vi "AudioOut Block Config Pane.vi"(6 "_SubPanelMessages":refnum<notifier>, 9 "_myEmbeddedToFrameEvent":T7, 10 "_myEmbedded.Exit":refnum<user-event>, 11 "-Property Bundle":cluster{"Name":string, "Value":variant}[](array[cluster])) -> (1 "_Connection Informations":T3, 2 "_Scripter Input":T9)   [LabVIEW 2021]
doc: "Writes values to one or more audio output channels on the NI myRIO. Use this Express VI to write multiple samples for each channel at one time."
uses:
  <vilib>/myRIO/Common/Express VI Framework/xctls/myRIO Channel List/myRIO Channel List.xctl
  <vilib>/myRIO/Common/Express VI Framework/typedefs/Config Pane to Framework Ref.ctl
  <vilib>/myRIO/Common/Express VI Framework/typedefs/Data Validate Ref.ctl
  <vilib>/myRIO/Common/Express VI Framework/typedefs/Scripter Input.ctl
  <vilib>/myRIO/Common/Express VI Framework/typedefs/WireThrough Terminal Names.ctl
  <vilib>/myRIO/Common/Express VI Framework/typedefs/Instrument Driver Method Descriptor Array.ctl
  <vilib>/myRIO/Common/Express VI Framework/typedefs/Instrument Driver Method Descriptor.ctl
  <vilib>/myRIO/Common/Express VI Framework/typedefs/Sub Panel Messages.ctl
  <vilib>/myRIO/Common/Express VI Framework/typedefs/Connection Informations.ctl
  <vilib>/myRIO/Common/Instrument Driver Framework/Utilities/typedefs/Channel Types.ctl
  <vilib>/myRIO/Common/Express VI Framework/vis/Express VI Framework Strings Global.vi
panel:
  in  "Sample Rate Unit":string="kHz"
  out "_learnMoreLatency":string="Gaps exist between sequential n samples generations. Learn more"
  out "_learnMoreFrequency":string="Detailed information about valid sample rates for this Express VI. Learn more"
  in  "Wait Until Done?":bool caption="Wait until done?"
  in  "_Validate":bool
  in  "Sample Rate:":dbl=1.0 caption="Sample rate:"
  in  "Name:":string="Audio output (n samples)" caption="Node name:"
  in  "Selected Channel List":T1[](xcontrol)=[{"Channel Name"=0, "Channel Alias"="", "Remove Channel"=FALSE, "Index"=0}, {"Channel Name"=1, "Channel Alias"="", "Remove Channel"=FALSE, "Index"=1}]
  in  "_Default Alias String":string
  in  "_VI Default Name (Edit and make value default)":string="Audio output (n samples)"
  in  "_WireThrough Info (Edit and make value default)":T4={"WireThrough Top In"="AudioOut (N Samples) Ref In", "WireThrough Bottom In"="error in (no error)", "WireThrough Top Out"="AudioOut (N Samples) Ref Out", "WireThrough Bottom Out"="error out"}
  in  "_Template Array (Edit and make value default)":T5=[{"Function Name"="Smart Open", "VI Path"=path "<vilib>/myRIO/Instrument Drivers/Onboard IO/AudioOut Block/vis", "Script"=TRUE, "Inputs"=[{"name"="Channel Names", "value"=variant, "Config Pane Only"=TRUE, "Build Array"=FALSE, "Bundle Cluster"=FALSE, "Show Term"=FALSE, "alias"=[], "Required Input"=FALSE}], "Outputs"=[], "VI Class"=enum."Open", "Controls Refs[]"=[], "Inline"=FALSE}, {"Function Name"="Open", "VI Path"=path "<vilib>/myRIO/Instrument Drivers/Onboard IO/AudioOut Block/vis", "Script"=FALSE, "Inputs"=[{"name"="Channel Names", "value"=variant, "Config Pane Only"=TRUE, "Build Array"=FALSE, "Bundle Cluster"=FALSE, "Show Term"=FALSE, "alias"=[], "Required Input"=FALSE}], "Outputs"=[], "VI Class"=enum."Open", "Controls Refs[]"=[], "Inline"=FALSE}, {"Function Name"="Write", "VI Path"=path "<vilib>/myRIO/Instrument Drivers/Onboard IO/AudioOut Block/vis", "Script"=TRUE, "Inputs"=[{"name"="Values", "value"=variant, "Config Pane Only"=FALSE, "Build Array"=TRUE, "Bundle Cluster"=FALSE, "Show Term"=TRUE, "alias"=[], "Required Input"=TRUE}, {"name"="Sample Rate [Hz]", "value"=variant, "Config Pane Only"=TRUE, "Build Array"=FALSE, "Bundle Cluster"=FALSE, "Show Term"=FALSE, "alias"=[], "Required Input"=FALSE}, {"name"="Wait Until Done?", "value"=variant, "Config Pane Only"=TRUE, "Build Array"=FALSE, "Bundle Cluster"=FALSE, "Show Term"=FALSE, "alias"=[], "Required Input"=FALSE}], "Outputs"=[], "VI Class"=enum."Data", "Controls Refs[]"=[], "Inline"=FALSE}, {"Function Name"="Close", "VI Path"=path "<vilib>/myRIO/Instrument Drivers/Onboard IO/AudioOut Block/vis", "Script"=FALSE, "Inputs"=[], "Outputs"=[], "VI Class"=enum."Close", "Controls Refs[]"=[], "Inline"=FALSE}]
  in  "_Test Close":bool
  # "User Visible Area"
  # "NOTE: Tab Order has been set\nfor this Front Panel.\n1. Name: (string control)\n2. Add Channel (button)\n3. Selected Channel List (array)\n\nAll other controls are excluded \nfrom Tabbing order\n\nTo exlude a control from context\nhelp prefix its label text with a '-'"
  # "kHz"
  # "This Express VI waits until the write operation completes."
  # "Gap:"
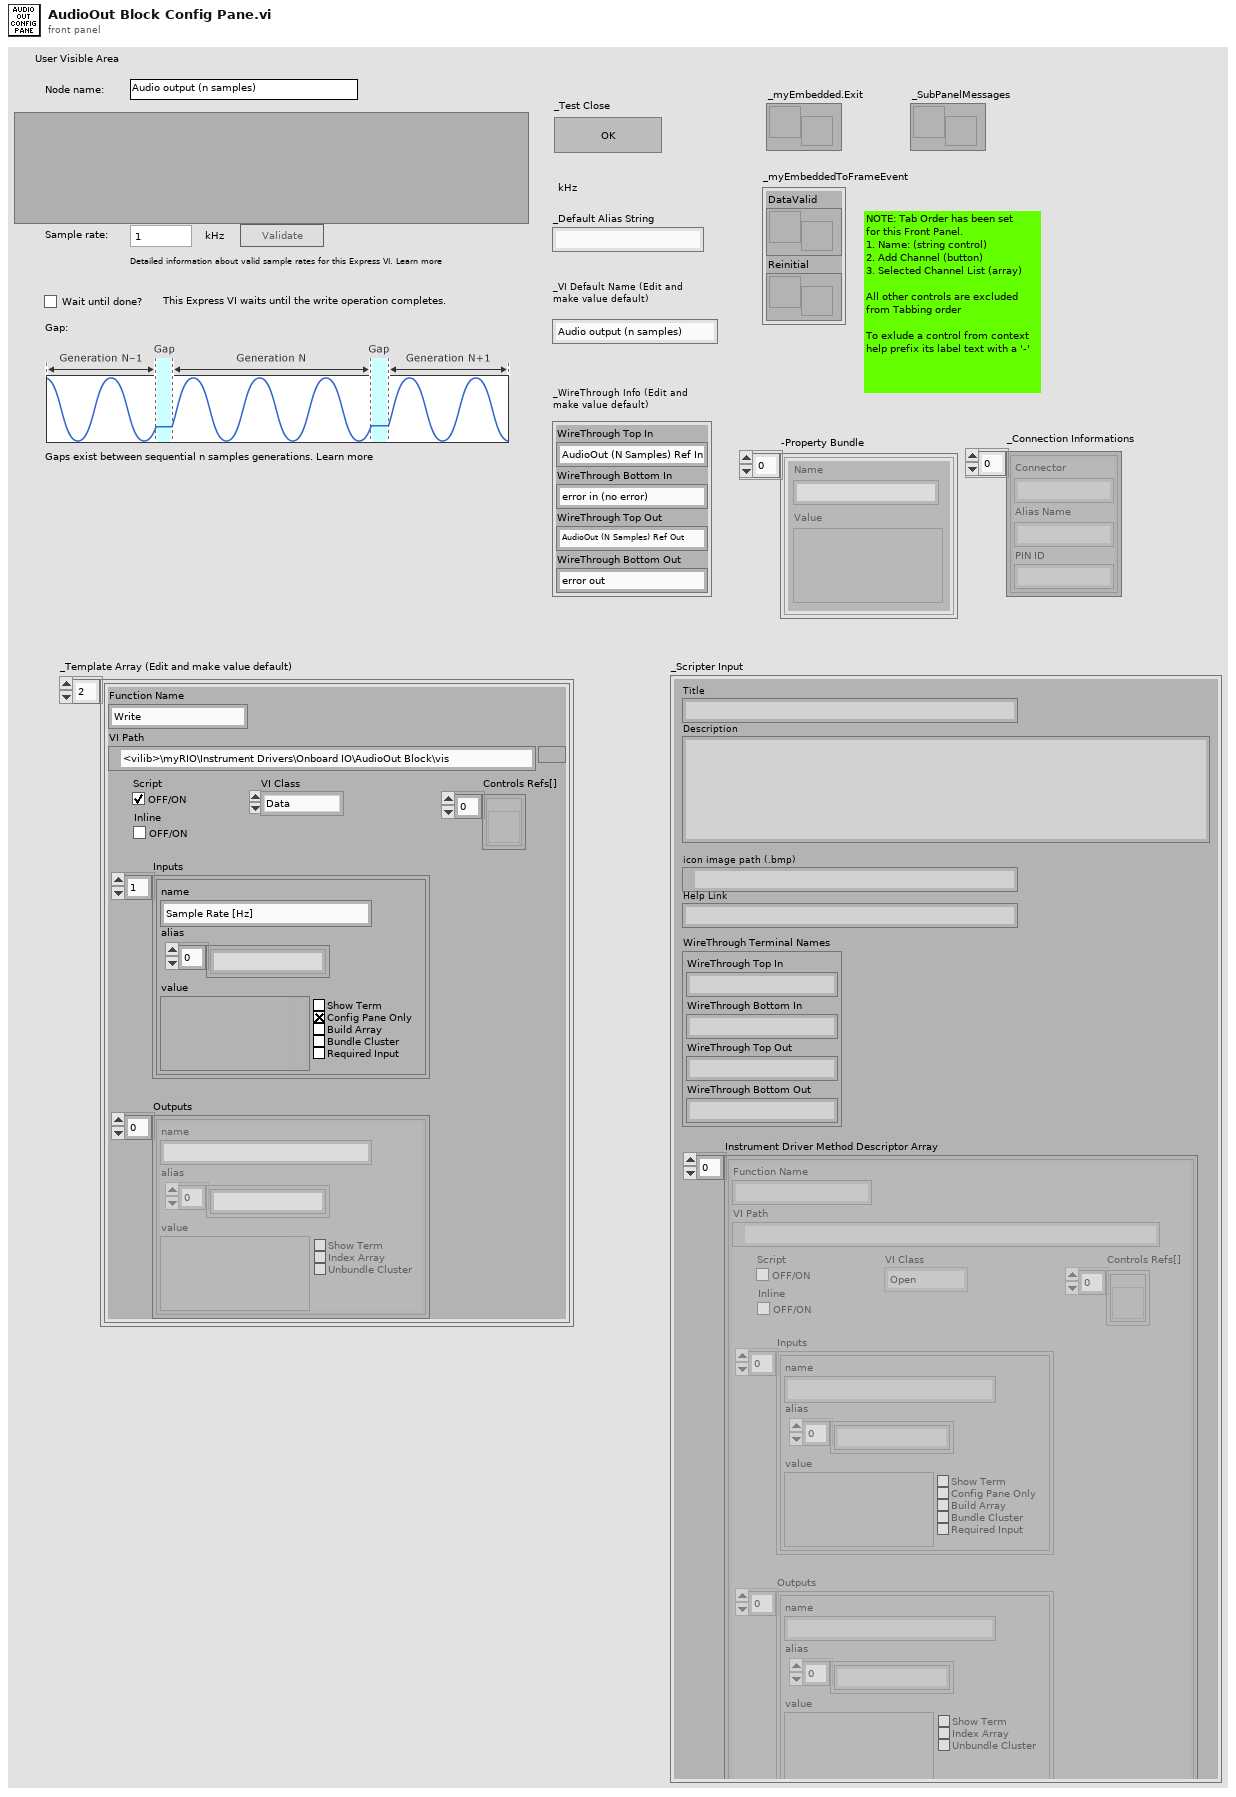
[diagram p1: front panel]
types:
  T1 = typedef "myRIO Channel List.xctl/Channel Data.ctl" = cluster{"Channel Name":u16, "Channel Alias":string, "Remove Channel":T2, "Index":i32}
  T2 = typedef "myRIO Channel List.xctl/Remove Channel.ctl" = bool
  T3 = typedef "Connection Informations.ctl" = cluster{"Connector":string, "Alias Name":string, "PIN ID":string}[]
  T4 = typedef "WireThrough Terminal Names.ctl" = cluster{"WireThrough Top In":string, "WireThrough Bottom In":string, "WireThrough Top Out":string, "WireThrough Bottom Out":string}
  T5 = typedef "Instrument Driver Method Descriptor Array.ctl" = T6[]
  T6 = typedef "Instrument Driver Method Descriptor.ctl" = cluster{"Function Name":string, "VI Path":path, "Script":bool, "Inputs":cluster{"name":string, "value":variant, "Config Pane Only":bool, "Build Array":bool, "Bundle Cluster":bool, "Show Term":bool, "alias":string[], "Required Input":bool}[], "Outputs":cluster{"name":string, "value":variant, "Show Term":bool, "Index Array":bool, "Unbundle Cluster":bool, "alias":string[]}[], "VI Class":enum16{"Open", "Configure", "Data", "Manage", "Close"}, "Controls Refs[]":refnum<vi>[], "Inline":bool}
  T7 = typedef "Config Pane to Framework Ref.ctl" = cluster{"DataValid":T8, "Reinitial":refnum<user-event>}
  T8 = typedef "Data Validate Ref.ctl" = refnum<user-event>
  T9 = typedef "Scripter Input.ctl" = cluster{"Title":string, "Description":string, "icon image path (.bmp)":path, "Help Link":string, "WireThrough Terminal Names":T4, "Instrument Driver Method Descriptor Array":T5}
  T10 = typedef "Channel Types.ctl" = enum32{"Unknown", "AI", "AO", "DIO - DI", "DIO", "DIO - DO", "I2C", "PWM", "Encoder", "SPI", "UART", "Accelerometer", "DIO - LED", "DIO - Button", "AI (N Samples)", "AudioIn (N Samples)", "AO (N Samples)", "AudioOut (N Samples)", "DI (N Samples)", "DO (N Samples)", "AI IRQ", "DI IRQ", "Timer IRQ", "RSL", "Relay", "CAN", "AI (Continuous)", "AO (Continuous)"}
  T11 = typedef "Channel Info.ctl" = cluster{"Channel Name":string, "Alias":string, "Used?":bool, "Not Support?":bool, "Property Bundle":cluster{"Name":string, "Value":variant}[]}
  T12 = typedef "Sub Panel Messages.ctl" = enum16{"Initialized"}
  T13 = enum8{"Enabled", "Disabled", "Disabled and Grayed Out"}
  T14 = cluster{"Connector":string, "Alias Name":string, "PIN ID":string}[]
  T15 = cluster{"name":string, "value":variant, "Config Pane Only":bool, "Build Array":bool, "Bundle Cluster":bool, "Show Term":bool, "alias":string[], "Required Input":bool}[]
  T16 = cluster{"name":string, "value":variant, "Config Pane Only":bool, "Build Array":bool, "Bundle Cluster":bool, "Show Term":bool, "alias":string[], "Required Input":bool}
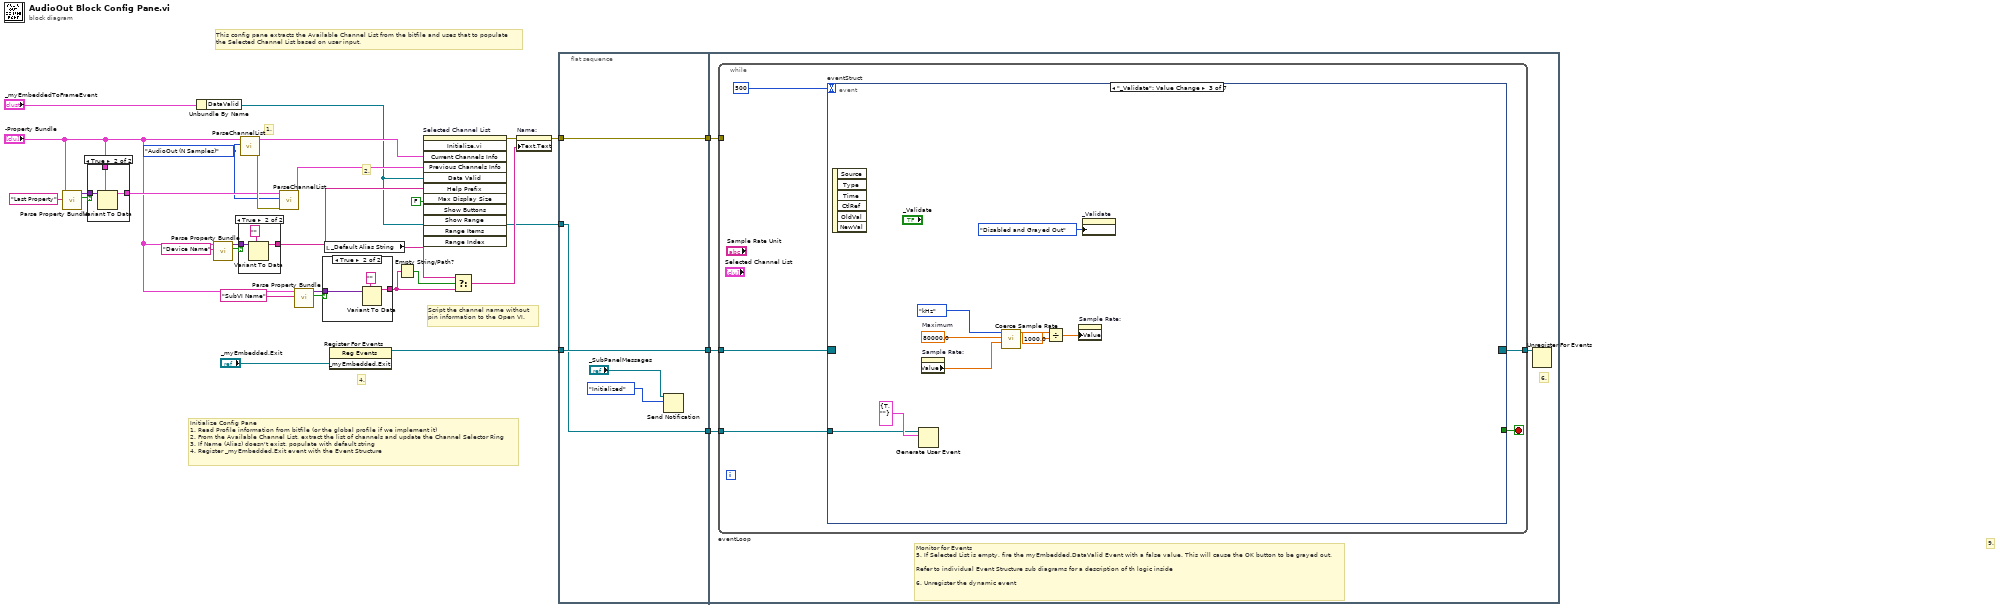
[diagram p0: block diagram]
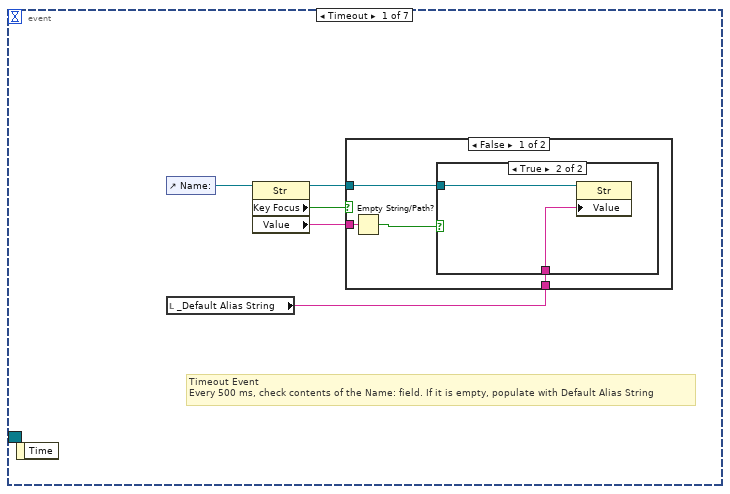
[diagram p2: hidden frame]
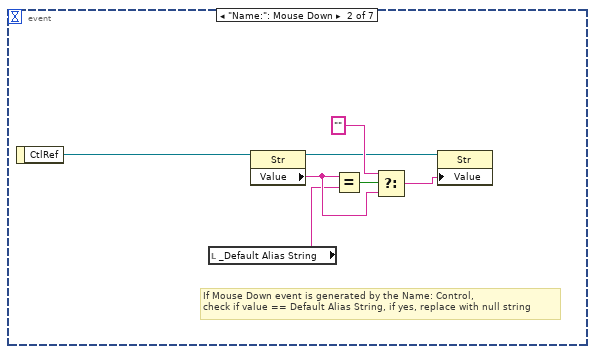
[diagram p5: hidden frame]
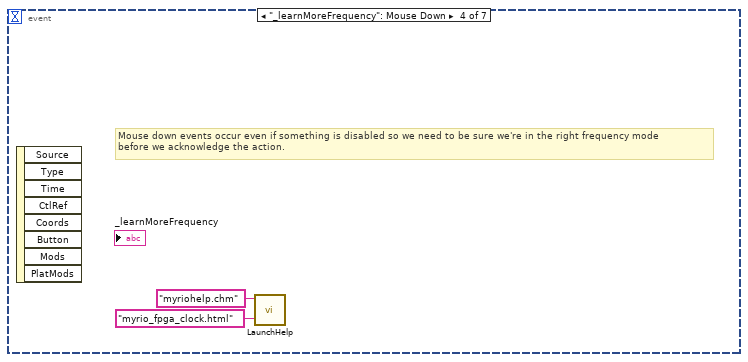
[diagram p6: hidden frame]
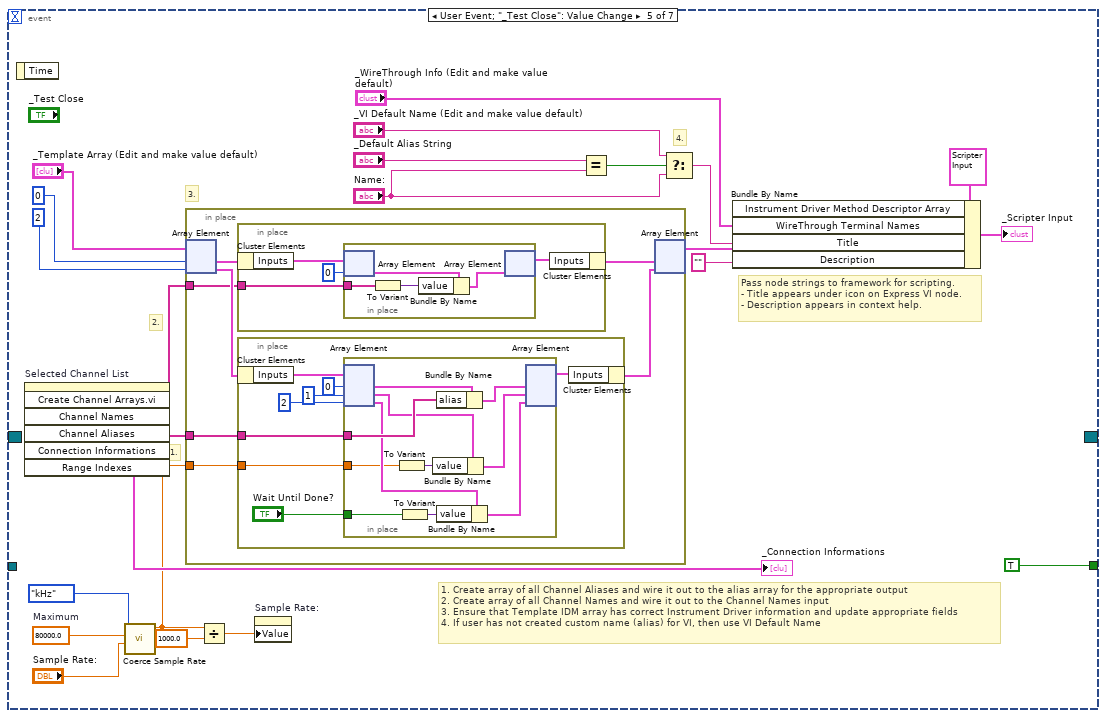
[diagram p7: hidden frame]
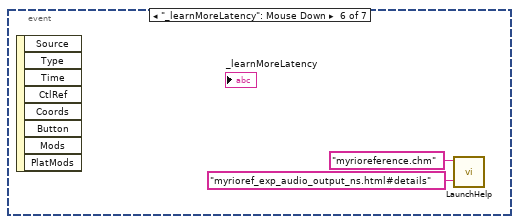
[diagram p8: hidden frame]
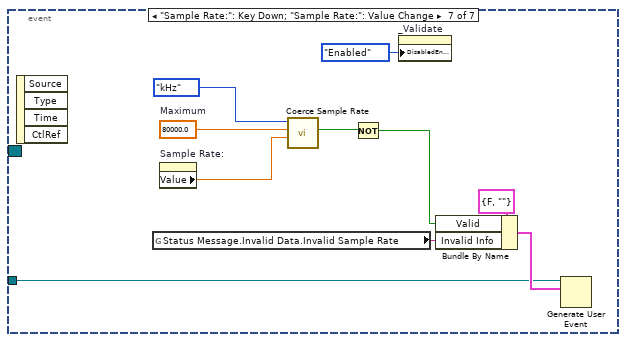
[diagram p9: hidden frame]
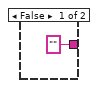
[diagram p12: hidden frame]
diagram:
  w10 = Channel_Types."AudioOut (N Samples)" ("Channel to Read")
  # "2."
  # "1."
  # "Script the channel name without pin information to the Open VI."
  # "This config pane extracts the Available Channel List from the bitfile and uses that to populate\nthe Selected Channel List based on user input."
  # "9."
  # "4."
  # "3."
  # "Initialize Config Pane\n1. Read Profile information from bitfile (or the global profile if we implement it)\n2. From the Available Channel List, extract the list of channels and update the Channel Selector Ring\n3. If Name (Alias) doesn't exist, populate with default string\n4. Register _myEmbedded.Exit event with the Event Structure"
  n1 = call <vilib>:"Parse Property Bundle.vi"("Name"="Last Property", "Property Bundle"="-Property Bundle") -> ("Found?"=w15:bool, "Value"=w16:variant)  [unwired: 8 in]
  n2 = case shown="True" w15 {
    tunnel: w16 -> [_ w33]
    tunnel: [_ w32] -> w13
    tunnel: "-Property Bundle" -> [_ w31]
    frame False {
    }
    frame True {
      n3 = Variant To Data(type=w31, Variant=w33) -> (data=w32:cluster{"Name":string, "Value":variant}[])  [unwired: 1 in, 1 out]
    }
  }
  n4 = Unbundle By Name("_myEmbeddedToFrameEvent") -> ("DataValid"=w2:T8)
  n5 = call <vilib>:"Parse Property Bundle.vi"("Name"="Device Name", "Property Bundle"="-Property Bundle") -> ("Found?"=w9:bool, "Value"=w8:variant)  [unwired: 8 in]
  n6 = case shown="True" w9 {
    tunnel: w8 -> [_ w36]
    tunnel: [_ w35] -> w5
    frame False {
    }
    frame True {
      n7 = Variant To Data(type="", Variant=w36) -> (data=w35:string)  [unwired: 1 in, 1 out]
    }
  }
  n8 = call <vilib>:"ParseChannelList.vi"("Channel to Read"=w10, "_Property Bundle"="-Property Bundle") -> ("error out"=w14:errorcluster, "Channel List Out"=w20:T11[])  [unwired: 7 in, 1 out]
  n9 = call <vilib>:"ParseChannelList.vi"("error in (no error)"=w14, "Channel to Read"=w10, "_Property Bundle"=w13) -> ("Channel List Out"=w12:T11[])  [unwired: 6 in, 2 out]
  n10 = call <vilib>:"Parse Property Bundle.vi"("Name"="SubVI Name", "Property Bundle"="-Property Bundle") -> ("Found?"=w24:bool, "Value"=w23:variant)  [unwired: 8 in]
  n11 = case shown="True" w24 {
    tunnel: w23 -> [_ w40]
    tunnel: ["" ("Name") w38] -> w22
    frame False {
    }
    frame True {
      n12 = Variant To Data(type="" ("Name"), Variant=w40) -> (data=w38:string)  [unwired: 1 in, 1 out]
    }
  }
  n13 = local read "_Default Alias String"() -> (w19:string)
  n14 = register-events("_myEmbedded.Exit") -> (reference out=w30:refnum<event-registration>)  [unwired: 2 in, 1 out]
  n15 = Empty String/Path?(string/path=w22) -> (empty?=w28:bool)
  n16 = invoke on="Selected Channel List" class="myRIO Channel List (strict)" method="Initialize.vi"("Current Channels Info"=w20, "Previous Channels Info"=w12, "Data Valid"=w2, "Help Prefix"=w5, "Show Buttons"=FALSE) -> (error out=w21:errorcluster)  [unwired: 7 in, 11 out]
  n17 = Select(t=w19, s=w28, f=w22) -> (s? t:f=w27:string)
  n18 = property on="Name:" class="Str"(error in=w21, "Text.Text"=w27) -> (error out=w26:errorcluster)  [unwired: 1 in, 1 out]
  n19 = flat-sequence {
    tunnel: w26 -> [w44]
    tunnel: w30 -> [w45]
    tunnel: [w45] -> w4
    tunnel: [w44] -> w3
    tunnel: w2 -> [w41]
    tunnel: [w41] -> w1
    tunnel: w4 -> [w49]
    tunnel: w3 -> [w47]
    tunnel: w1 -> [w46]
    frame #0 {
      n20 = Send Notification(notification=Sub_Panel_Messages."Initialized", notifier="_SubPanelMessages") -> ()  [unwired: 1 in, 2 out]
    }
    frame #1 {
      # "6."
      # "Monitor for Events\n5. If Selected List is empty, fire the myEmbedded.DataValid Event with a false value. This will cause the OK button to be grayed out.\n\nRefer to individual Event Structure sub diagrams for a description of th logic inside\n\n6. Unregister the dynamic event"
      n21 = while "eventLoop" {
        tunnel: w49 -> [w53]
        tunnel: [w52] -> w48
        tunnel: w47 -> [_]
        tunnel: w46 -> [w50]
        stop <- w54 stop-if-true
        n22 = event "eventStruct" shown="[2] \"_Validate\": Value Change" {
          selector: w53 -> [_ _ _ _ _ _ _]
          dyn-events: [_ _ _ _ _ _ _] -> w52
          timeout: 500 -> [_ _ _ _ _ _ _]
          tunnel: [_ _ _ _ TRUE ("_Test Close") _ _] -> w54
          tunnel: w50 -> [_ _ w73 _ _ _ w143]
          event Timeout {
            # "Timeout Event\nEvery 500 ms, check contents of the Name: field. If it is empty, populate with Default Alias String"
            n23 = event-data() -> ()  [unwired: 1 in, 1 out]
            n24 = control-ref of="Name:"() -> (w57:refnum<vi>)
            n25 = local read "_Default Alias String"() -> (w55:string)
            n26 = property on="Property Node" class="Str"(reference=w57) -> (reference out=w56:refnum<vi>, "Key Focus"=w58:bool, "Value"=w59:string)  [unwired: 1 in, 1 out]
            n27 = case shown="False" w58 {
              tunnel: w59 -> [w63 _]
              tunnel: w56 -> [w61 _]
              tunnel: w55 -> [w60 _]
              frame False {
                n28 = Empty String/Path?(string/path=w63) -> (empty?=w62:bool)
                n29 = case shown="True" w62 {
                  tunnel: w61 -> [_ w65]
                  tunnel: w60 -> [_ w64]
                  frame False {
                  }
                  frame True {
                    n30 = property on="Property Node" class="Str"(reference=w65, "Value"=w64) -> ()  [unwired: 1 in, 2 out]
                  }
                }
              }
              frame True {
              }
            }
          }
          event "Name:": Mouse Down {
            # "If Mouse Down event is generated by the Name: Control,\ncheck if value == Default Alias String, if yes, replace with null string"
            n31 = event-data() -> ("CtlRef"=w72:refnum<vi>)  [unwired: 1 in]
            n32 = local read "_Default Alias String"() -> (w66:string)
            n33 = property class="Str"(reference=w72) -> (reference out=w68:refnum<vi>, "Value"=w67:string)  [unwired: 1 in, 1 out]
            n34 = Equal?(x=w67, y=w66) -> (x = y?=w71:bool)
            n35 = Select(t="", s=w71, f=w67) -> (s? t:f=w69:string)
            n36 = property class="Str"(reference=w68, "Value"=w69) -> ()  [unwired: 1 in, 2 out]
          }
          event "_Validate": Value Change {
            w81 = 80000.0  # Maximum
            n37 = event-data() -> ()  [unwired: 1 in, 6 out]
            n38 = Generate User Event(user event=w73, event data cluster=cluster{"Valid":bool, "Invalid Info":string} {"Valid"=TRUE, "Invalid Info"=""} ("event data")) -> ()  [unwired: 2 in, 2 out]
            n39 = property on="Sample Rate:" class="DigNum (strict)"() -> ("Value"=w80:dbl)  [unwired: 2 in, 2 out]
            n40 = call <vilib>:"Coerce Sample Rate.vi"("Sample Rate:"=w80, "Maximum"=w81, "Sample Rate Unit"=enum16{"Hz", "kHz", "MHz"}."kHz") -> ("Actual Sample Rate (s)"=w77:dbl)  [unwired: 7 in, 1 out]
            n41 = Divide(x=w77, y=1000.0) -> (x/y=w75:dbl)
            n42 = property on="Sample Rate:" class="DigNum (strict)"("Value"=w75) -> ()  [unwired: 2 in, 2 out]
            n43 = property on="_Validate" class="Bool"("DisabledEnum"=T13."Disabled and Grayed Out" ("Disabled")) -> ()  [unwired: 2 in, 2 out]
          }
          event "_learnMoreFrequency": Mouse Down {
            # "Mouse down events occur even if something is disabled so we need to be sure we're in the right frequency mode\nbefore we acknowledge the action."
            n44 = event-data() -> ()  [unwired: 1 in, 8 out]
            n45 = call <vilib>:"LaunchHelp.vi"("Help Topic"="myrio_fpga_clock.html", "Help File"="myriohelp.chm") -> ()  [unwired: 10 in]
          }
          event User Event; "_Test Close": Value Change {
            w92 = 80000.0  # Maximum
            # "2."
            # "1."
            # "1. Create array of all Channel Aliases and wire it out to the alias array for the appropriate output\n2. Create array of all Channel Names and wire it out to the Channel Names input\n3. Ensure that Template IDM array has correct Instrument Driver information and update appropriate fields\n4. If user has not created custom name (alias) for VI, then use VI Default Name"
            # "4."
            # "3."
            # "Pass node strings to framework for scripting.\n- Title appears under icon on Express VI node.\n- Description appears in context help."
            n46 = event-data() -> ()  [unwired: 1 in, 1 out]
            n47 = invoke on="Selected Channel List" class="myRIO Channel List (strict)" method="Create Channel Arrays.vi"() -> ("Channel Names"=w90:string[], "Channel Aliases"=w89:string[], "Connection Informations"=→"_Connection Informations":T14)  [unwired: 7 in, 4 out]
            n48 = call <vilib>:"Coerce Sample Rate.vi"("Sample Rate:"="Sample Rate:", "Maximum"=w92, "Sample Rate Unit"=enum16{"Hz", "kHz", "MHz"}."kHz") -> ("Actual Sample Rate (s)"=w86:dbl)  [unwired: 7 in, 1 out]
            n49 = in-place {
              in-place-border: w90 -> [w109]
              in-place-border: w89 -> [w108]
              in-place-border: w86 -> [w107]
              n50 = in-place-array #1("_Template Array (Edit and make value default)", 0, 2) -> (w113:T6, w111:T6)
              n51 = in-place {
                in-place-border: w109 -> [w135]
                n52 = in-place-cluster #2(w113) -> ("Inputs"=w136:T15)
                n53 = in-place {
                  in-place-border: w135 -> [w137]
                  n54 = in-place-array #3(w136, 0) -> (w140:T16)
                  n55 = To Variant(anything=w137) -> (Variant=w138:variant)
                  n56 = Bundle By Name(cluster=w140, "value"=w138) -> (w139:T16)
                  n57 = in-place-array #3(w139) -> (w134:T15)  [unwired: 1 out]
                }
                n58 = in-place-cluster #2("Inputs"=w134) -> (w112:T6)
              }
              n59 = in-place {
                in-place-border: w108 -> [w120]
                in-place-border: w107 -> [w115]
                n60 = in-place-cluster #4(w111) -> ("Inputs"=w121:T15)
                n61 = in-place {
                  in-place-border: w120 -> [w130]
                  in-place-border: w115 -> [w125]
                  in-place-border: "Wait Until Done?" -> [w124]
                  n62 = in-place-array #5(w121, 0, 1, 2) -> (w132:T16, w129:T16, w128:T16)
                  n63 = To Variant(anything=w125) -> (Variant=w127:variant)
                  n64 = To Variant(anything=w124) -> (Variant=w126:variant)
                  n65 = Bundle By Name(cluster=w129, "value"=w127) -> (w123:T16)
                  n66 = Bundle By Name(cluster=w132, "alias"=w130) -> (w131:T16)
                  n67 = Bundle By Name(cluster=w128, "value"=w126) -> (w122:T16)
                  n68 = in-place-array #5(w131, w123, w122) -> (w119:T15)  [unwired: 3 out]
                }
                n69 = in-place-cluster #4("Inputs"=w119) -> (w110:T6)
              }
              n70 = in-place-array #1(w112, w110) -> (w104:T5)  [unwired: 2 out]
            }
            n71 = Divide(x=w86, y=1000.0) -> (x/y=w84:dbl)
            n72 = property on="Sample Rate:" class="DigNum (strict)"("Value"=w84) -> ()  [unwired: 2 in, 2 out]
            n73 = Equal?(x="_Default Alias String", y="Name:") -> (x = y?=w96:bool)
            n74 = Select(t="_VI Default Name (Edit and make value default)", s=w96, f="Name:") -> (s? t:f=w94:string)
            n75 = Bundle By Name(cluster=T9 {"Title"="", "Description"="", "icon image path (.bmp)"=path "", "Help Link"="", "WireThrough Terminal Names"={"WireThrough Top In"="", "WireThrough Bottom In"="", "WireThrough Top Out"="", "WireThrough Bottom Out"=""}, "Instrument Driver Method Descriptor Array"=[]} ("Scripter Input"), "Instrument Driver Method Descriptor Array"=w104, "WireThrough Terminal Names"="_WireThrough Info (Edit and make value default)", "Title"=w94, "Description"="" ("Title")) -> (→"_Scripter Input":T9)
          }
          event "_learnMoreLatency": Mouse Down {
            n76 = event-data() -> ()  [unwired: 1 in, 8 out]
            n77 = call <vilib>:"LaunchHelp.vi"("Help Topic"="myrioref_exp_audio_output_ns.html#details", "Help File"="myrioreference.chm") -> ()  [unwired: 10 in]
          }
          event "Sample Rate:": Key Down; "Sample Rate:": Value Change {
            w147 = 80000.0  # Maximum
            n78 = event-data() -> ()  [unwired: 1 in, 4 out]
            n79 = global read "Express VI Framework Strings Global.vi" "Status Message.Invalid Data.Invalid Sample Rate"() -> (w149:string)
            n80 = property on="Sample Rate:" class="DigNum (strict)"() -> ("Value"=w146:dbl)  [unwired: 2 in, 2 out]
            n81 = call <vilib>:"Coerce Sample Rate.vi"("Sample Rate:"=w146, "Maximum"=w147, "Sample Rate Unit"=enum16{"Hz", "kHz", "MHz"}."kHz") -> ("Coercion needed?"=w144:bool)  [unwired: 7 in, 1 out]
            n82 = Not(x=w144) -> (.not. x?=w148:bool)
            n83 = property on="_Validate" class="Bool"("DisabledEnum"=T13."Enabled" ("Disabled")) -> ()  [unwired: 2 in, 2 out]
            n84 = Bundle By Name(cluster=cluster{"Valid":bool, "Invalid Info":string} {"Valid"=FALSE, "Invalid Info"=""} ("event data"), "Valid"=w148, "Invalid Info"=w149) -> (w150:cluster{"Valid":bool, "Invalid Info":string})
            n85 = Generate User Event(user event=w143, event data cluster=w150) -> ()  [unwired: 2 in, 2 out]
          }
        }
      }
      n86 = Unregister For Events(event registration refnum=w48) -> ()  [unwired: 1 in, 1 out]
    }
  }
